vi "All Off.vi"(8 "error in (no error)":errorcluster, 11 "VISA resource name":refnum<visa-resource-name>) -> (0 "error out 2":errorcluster, 3 "VISA resource name out":refnum<visa-resource-name>)   [LabVIEW 2012, in "Fluke 2625A.lvlib"]
uses:
  <instrlib>/Fluke 2625A/Fluke 2625A.lvlib
panel:
  out "All sent strings":string[](array[string])
  out "read buffer":string
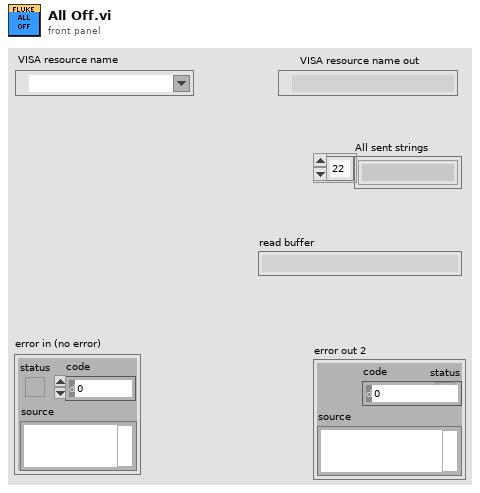
[diagram p1: front panel]
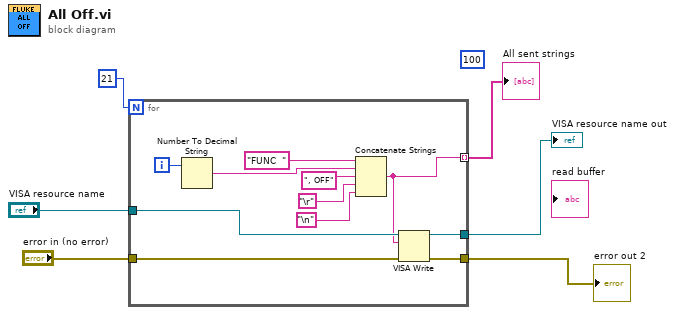
[diagram p0: block diagram]
diagram:
  (unwired) u32 100 ("byte count")
  n1 = for {
    N: 21 -> [_]
    tunnel: [w17] -> w1
    tunnel: [w16] -> w2
    tunnel: "VISA resource name" -> [w14]
    tunnel: "error in (no error)" -> [w13]
    tunnel: [w12] -> w3 mode=indexing
    i -> [w11]
    n2 = Number To Decimal String(number=w11) -> (decimal integer string=w15:string)  [unwired: 1 in]
    n3 = Concatenate Strings("FUNC  " ("string"), w15, ", OFF" ("string"), "\r", "\n") -> (w12:string)
    n4 = VISA Write(VISA resource name=w14, write buffer=w12, error in (no error)=w13) -> (VISA resource name out=w16:refnum<visa-resource-name>, error out=w17:errorcluster)  [unwired: 1 out]
  }
  "VISA resource name out" <- w2
  "All sent strings" <- w3
  "error out 2" <- w1
